vi "Control Loop State 2 Flags.vi"(0 "L1 Ctrl Loop State":T1) -> (1 "Controlled":bool, 2 "Autobalanced":bool)   [LabVIEW 2009]
uses:
  Control Loop State.ctl
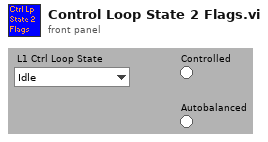
[diagram p1: front panel]
types:
  T1 = typedef "Control Loop State.ctl" = enum16{"Idle", "Off", "Reset Autobalancing", "Autobalancing", "Set Command", "Ready for Control", "On"}
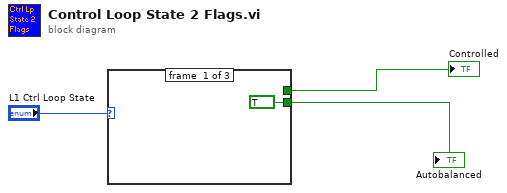
[diagram p0: block diagram]
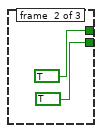
[diagram p2: hidden frame]
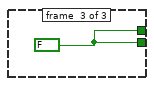
[diagram p3: hidden frame]
diagram:
  n1 = case shown="\"Idle\", Default" "L1 Ctrl Loop State" {
    tunnel: [TRUE TRUE w7] -> w2
    tunnel: [_ TRUE w7] -> w3
    frame #0 {
    }
    frame #1 {
    }
    frame #2 {
      w7 = FALSE
    }
  }
  "Controlled" <- w3
  "Autobalanced" <- w2
